vi "PicoLog_DATA_2.vi"(1 "k m":i32[](array[numeric])=[2, 0, 2, 0, 0, 0, 6, 0, 0, 0, 0, 0, 0, 0, 0, 0] min=0 max=6 step=1, 5 "noOfChannels":i16, 7 "handle":i16, 8 "sampleInterval_ms":dbl) -> (4 "x*y":dbl[](array[numeric]), 6 "handle":i16)   [LabVIEW 2014]
uses:
  picohrdl.dll
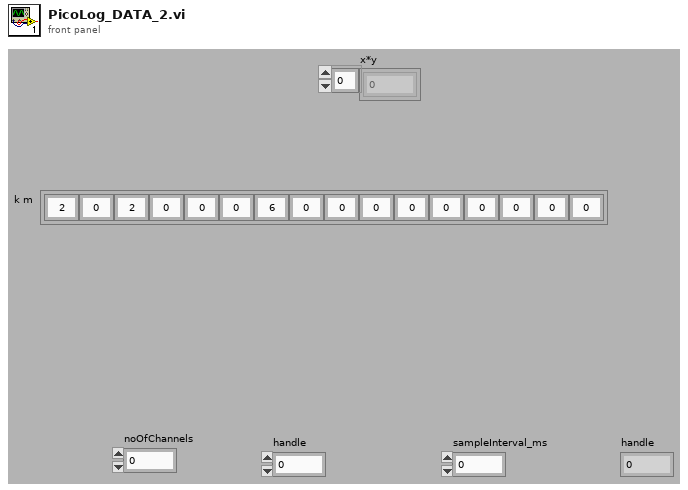
[diagram p1: front panel]
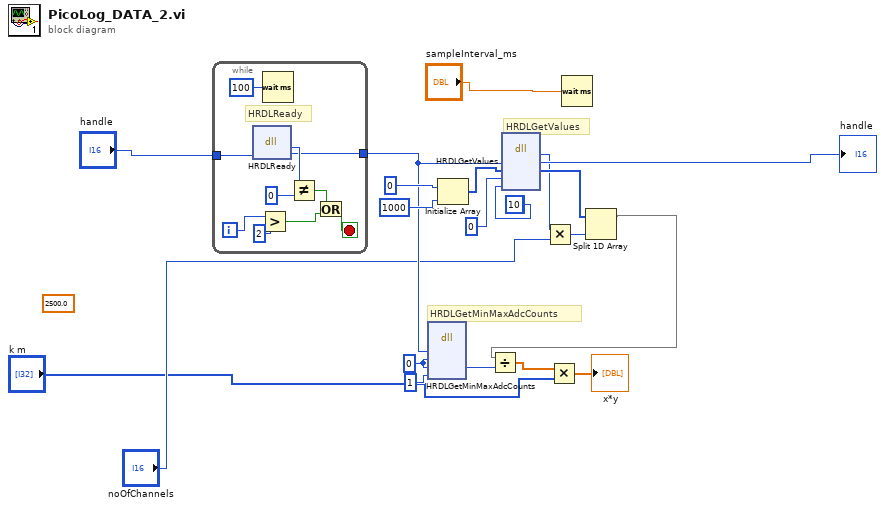
[diagram p0: block diagram]
diagram:
  (unwired) 2500.0
  w13 = 0 ("maxAdc")
  (unwired) 10 ("noOfValues")
  # "HRDLGetMinMaxAdcCounts"
  # "HRDLGetValues"
  n1 = while {
    tunnel: "handle" -> [w28]
    tunnel: [w27] -> w5
    i -> [w25]
    stop <- w23 stop-if-true
    # "HRDLReady"
    n2 = dll-call lib="PicoHRDL.dll" fn="HRDLReady"("handle"=w28) -> ("ready"=w30:i16, "handle"=w27:i16)  [unwired: 3 in, 2 out]
    n3 = Greater?(x=w25, y=2) -> (0:w21:bool)
    n4 = Wait (ms)(milliseconds to wait=u32 100) -> ()  [unwired: 1 out]
    n5 = Not Equal?(x=w30, y=i16 0) -> (x != y?=w22:bool)
    n6 = Or(x=w22, y=w21) -> (x .or. y?=w23:bool)
  }
  n7 = dll-call lib="PicoHRDL.dll" fn="HRDLGetMinMaxAdcCounts"("handle"=w5, "minAdc"=w13, "maxAdc"=w13, "channel"=i16 1) -> ("maxAdc"=w8:i32)  [unwired: 7 in, 2 out]
  n8 = Initialize Array(0 ("element"), 1000 ("dimension size")) -> (w20:i32[])
  n9 = dll-call lib="PicoHRDL.dll" fn="HRDLGetValues"("handle"=w5, "values"=w20, "overflow"=i16 0, "noOfValues"=10) -> ("noValuesPerChan"=w9:i32, "handle"=→"handle":i16, "values"=w11:i32[])  [unwired: 5 in, 2 out]
  n10 = Multiply(x=w9, y="noOfChannels") -> (x*y=w10:i32)
  n11 = Wait (ms)(milliseconds to wait="sampleInterval_ms") -> ()  [unwired: 1 out]
  n12 = Split 1D Array(array=w11, index=w10) -> (first subarray=w3:i32[])  [unwired: 1 out]
  n13 = Divide(x=w3, y=w8) -> (x/y=w12:dbl[])
  n14 = Multiply(x=w12, y="k m") -> (x*y=→"x*y":dbl[])
